vi "Zatwierdzenie ustalonego zakresu.vi"(11 "Skalowanie in":T1) -> (2 "Dł. piksela[m]":dbl caption="Długość piksela w metrach", 3 "Skalowanie out":T1)   [LabVIEW 2015, in "Biblioteka moduł map v3.lvlib" / "Pomocnicze.lvlib"]
doc: "Zadaniem pliku jest ustawienie długości piksela w metrach, którą można wyznaczyć na podstawie:\n1. Odległości podanej w metrach pomiędzy dwoma ustawionymi znacznikami.\n2. Na podstawie współrzędnych geograficznych wprowadzonych dla każdego znacznika z osobna.\nPo użyciu VI w \"Skalowanie out\" ustawiana jest blokada znaczników."
uses:
  Pomocnicze.lvlib
  Matematyczne/Matematyczne.lvlib
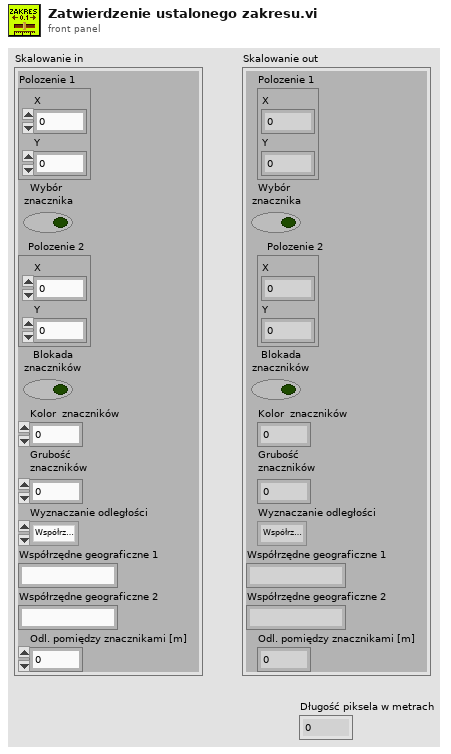
[diagram p1: front panel]
types:
  T1 = cluster{"Polozenie 1":cluster{"X":i32, "Y":i32}, "  Wybór \nznacznika":bool, "   Polozenie 2":cluster{"X":i32, "Y":i32}, "   Blokada \nznaczników":bool, "Kolor  znaczników":u32, "Grubość \nznaczników":u32, "Wyznaczanie odległości":enum16{"Współrzędne geograficzne", "Odległość pomiędzy znacznikami"}, "Współrzędne geograficzne 1":string, "Współrzędne geograficzne 2":string, "Odl. pomiędzy znacznikami [m]":dbl}
  T2 = enum16{"Współrzędne geograficzne", "Odległość pomiędzy znacznikami"}
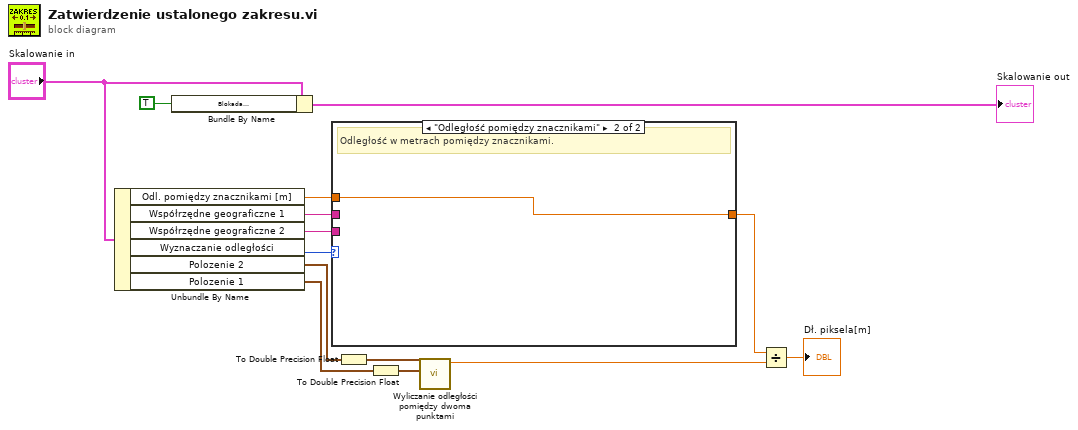
[diagram p0: block diagram]
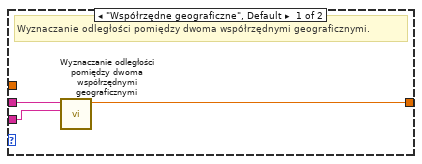
[diagram p2: hidden frame]
diagram:
  n1 = Unbundle By Name("Skalowanie in") -> ("Odl. pomiędzy znacznikami [m]"=w14:dbl, "Współrzędne geograficzne 1"=w8:string, "Współrzędne geograficzne 2"=w9:string, "Wyznaczanie odległości"=w10:T2, "Polozenie 2"=w4:cluster{"X":i32, "Y":i32}, "Polozenie 1"=w2:cluster{"X":i32, "Y":i32})
  n2 = Bundle By Name(cluster="Skalowanie in", "Blokada \nznaczników"=TRUE ("Blokada \nznaczników")) -> (→"Skalowanie out":T1)
  n3 = case shown="\"Odległość pomiędzy znacznikami\"" w10 {
    tunnel: [w17 w18] -> w7
    tunnel: w8 -> [w16 _]
    tunnel: w9 -> [w15 _]
    tunnel: w14 -> [_ w18]
    frame "Współrzędne geograficzne", Default {
      # "Wyznaczanie odległości pomiędzy dwoma współrzędnymi geograficznymi."
      n4 = call "Wyznaczanie odległości pomiędzy dwoma współrzędnymi geograficznymi.vi"("Współrzędne geograficzne in"=w15, "Współrzędne geograficzne 1"=w16) -> ("Numeric"=w17:dbl)  [unwired: 9 in]
    }
    frame "Odległość pomiędzy znacznikami" {
      # "Odległość w metrach pomiędzy znacznikami."
    }
  }
  n5 = To Double Precision Float(number=w4) -> (double precision float=w5:cluster{"X":dbl, "Y":dbl})
  n6 = To Double Precision Float(number=w2) -> (double precision float=w3:cluster{"X":dbl, "Y":dbl})
  n7 = call "Wyliczanie odległości pomiędzy dwoma punktami.vi"("Polozenie 1"=w3, "Polozenie in"=w5) -> ("Numeric"=w6:dbl)  [unwired: 9 in]
  n8 = Divide(x=w7, y=w6) -> (x/y=→"Dł. piksela[m]":dbl)
